vi "Delay And Channel Names_DG535.vi"(0 "Channel Array":refnum<vi>[](array[refnum])) -> (1 "Array":T1[](array[typedef]) min=-999.0 max=999.0 format="%+.12f", 2 "Array 2":string[](array[string]))   [LabVIEW 2013]
uses:
  GUI_DG645/DelayControl2.ctl
  Device Driver/DG645/subVIs/channels_TypDef.ctl
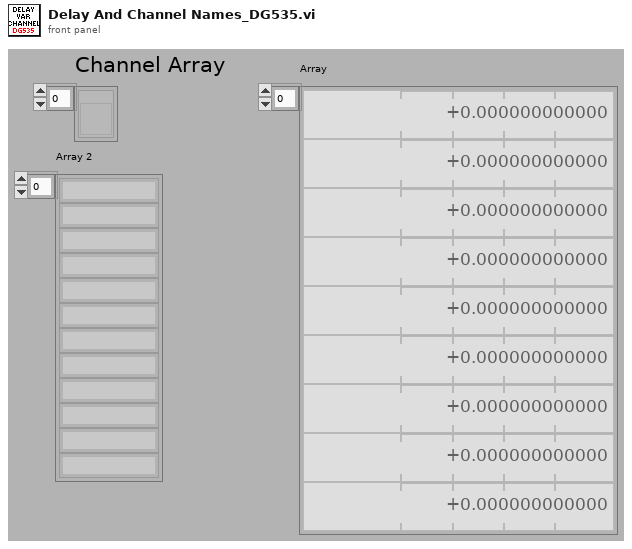
[diagram p1: front panel]
types:
  T1 = typedef "DelayControl2.ctl" = dbl
  T2 = typedef "channels_TypDef.ctl" = enum16{"T0", "T1", "A", "B", "C", "D", "E", "F", "G", "H"}
  T3 = typedef "channels_TypDef_DG535.ctl" = enum16{"T0", "A", "B", "C", "D"}
  T4 = cluster{"Channel":string, "reference":T3, "delay":T1}
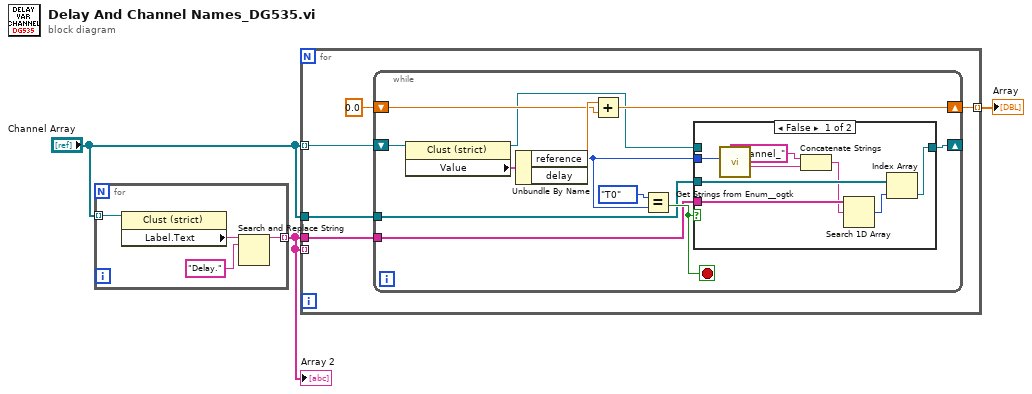
[diagram p0: block diagram]
diagram:
  n1 = for {
    tunnel: "Channel Array" -> [w7] mode=indexing
    tunnel: [w4] -> w1 mode=indexing
    n2 = property class="Clust (strict)"(reference=w7) -> ("Label.Text"=w6:string)  [unwired: 1 in, 2 out]
    n3 = Search and Replace String(input string=w6, search string="Delay.") -> (result string=w4:string)  [unwired: 6 in, 3 out]
  }
  "Array 2" <- w1
  n4 = for {
    tunnel: "Channel Array" -> [w10] mode=indexing
    tunnel: w1 -> [w12]
    tunnel: "Channel Array" -> [w11]
    tunnel: [w8] -> w2 mode=indexing
    tunnel: w1 -> [_] mode=indexing
    n5 = while {
      shift-right: [w20] -> w8
      shift-left: T1 0.0 ("Delay") -> [w21]
      shift-right: [w15] -> _
      shift-left: w10 -> [w13]
      tunnel: w12 -> [w17]
      tunnel: w11 -> [w16]
      stop <- w19 stop-if-true
      n6 = property class="Clust (strict)"(reference=w13) -> (reference out=w14:refnum<vi>, "Value"=w24:T4)  [unwired: 1 in, 1 out]
      n7 = Unbundle By Name(w24) -> ("reference"=w18:T3, "delay"=w22:T1)
      n8 = Add(x=w22, y=w21) -> (x+y=w20:T1)
      n9 = Equal?(x=channels_TypDef."T0" ("Linked"), y=w18) -> (x = y?=w19:bool)
      n10 = case shown="False" w19 {
        tunnel: w18 -> [w32 _]
        tunnel: w17 -> [w31 _]
        tunnel: w16 -> [w29 _]
        tunnel: [w28 w33] -> w15
        tunnel: w14 -> [_ w33]
        frame False {
          n11 = call <userlib>:"Get Strings from Enum__ogtk.vi"("Enum"=w32) -> ("String Value"=w26:string)  [unwired: 7 in, 3 out]
          n12 = Concatenate Strings("Channel_" ("string"), w26) -> (w25:string)
          n13 = Search 1D Array(1D array=w31, element=w25) -> (index of element=w30:i32)  [unwired: 1 in]
          n14 = Index Array(array=w29, index=w30) -> (element=w28:refnum<vi>)
        }
        frame True {
        }
      }
    }
  }
  "Array" <- w2
